vi "Command Settings.vi"() -> (5 "Command Settings":T1[](array[typedef])=[{"Enum"=enum."Connect Channel", "U8"=0, " Payload"=TRUE}, {"Enum"=enum."Force Channel", "U8"=0, " Payload"=FALSE}, {"Enum"=enum."Force Channel", "U8"=0, " Payload"=TRUE}, {"Enum"=enum."Add FIFO Pub", "U8"=0, " Payload"=TRUE}, {"Enum"=enum."Connect Channel", "U8"=0, " Payload"=TRUE}, {"Enum"=enum."Connect Channel", "U8"=0, " Payload"=FALSE}, {"Enum"=enum."Connect Channel", "U8"=0, " Payload"=TRUE}, {"Enum"=enum."Connect Channel", "U8"=0, " Payload"=FALSE}, {"Enum"=enum."Connect Channel", "U8"=0, " Payload"=FALSE}, {"Enum"=enum."Connect Channel", "U8"=0, " Payload"=FALSE}])   [LabVIEW 2021, in "ChanMngOOB_Rx.lvclass"]
uses:
  ChanMngOOB_Rx.lvclass
  Typedef/Command Setting Control.ctl
  Typedef/OOB ChnMng Commands.ctl
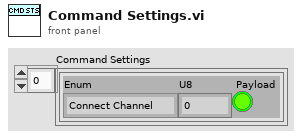
[diagram p1: front panel]
types:
  T1 = typedef "ChanMngOOB_Rx.lvclass/Command Setting Control.ctl" = cluster{"Enum":T2, "U8":u8, " Payload":bool}
  T2 = typedef "ChanMngOOB_Rx.lvclass/OOB ChnMng Commands.ctl" = enum8{"Connect Channel", "Force Channel", "Add FIFO Pub", "Remove FIFO Pub"}
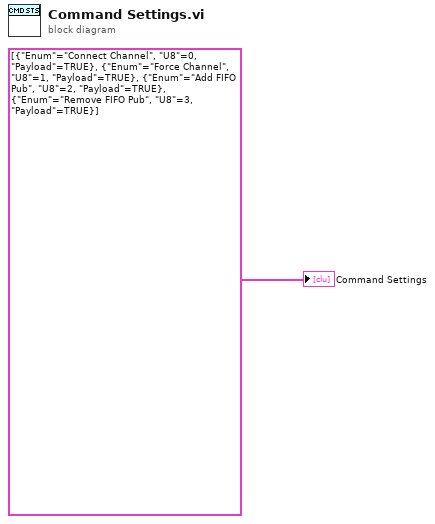
[diagram p0: block diagram]
diagram:
  "Command Settings" <- cluster{"Enum":T2, "U8":u8, "Payload":bool}[] [{"Enum"=enum."Connect Channel", "U8"=0, "Payload"=TRUE}, {"Enum"=enum."Force Channel", "U8"=1, "Payload"=TRUE}, {"Enum"=enum."Add FIFO Pub", "U8"=2, "Payload"=TRUE}, {"Enum"=enum."Remove FIFO Pub", "U8"=3, "Payload"=TRUE}]
